vi "Get Alias.vi"(8 "error in (no error)":errorcluster, 11 "Project Action in":refnum<class "Project Action.lvclass">) -> (0 "error out":errorcluster, 2 "Alias":string, 3 "Project Action out":refnum<class "Project Action.lvclass">)   [LabVIEW 2020, in "ProjectBuilder.lvlib" / "Project Action.lvclass"]
uses:
  Project Action.lvclass
  C:/Current projects/WS/LV32.2020..ProjectBuilder/Class/Action/Project Action/Project Action.lvclass
  C:/Current projects/WS/LV32.2020..ProjectBuilder/Interface/Project Action Interface/Project Action Interface.lvclass
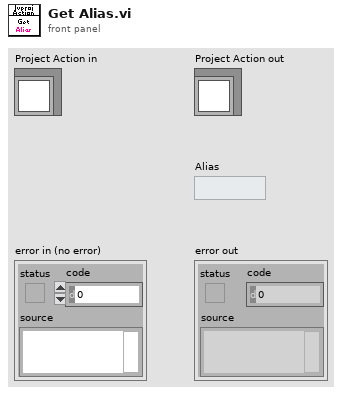
[diagram p1: front panel]
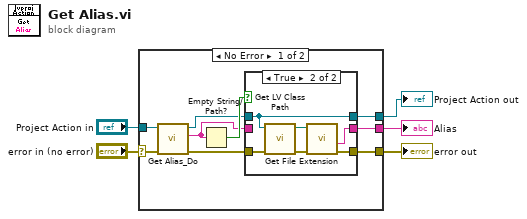
[diagram p0: block diagram]
diagram:
  n1 = case shown="No Error" "error in (no error)" {
    selector: "error in (no error)" -> [w14 w25]
    tunnel: [w7 w25] -> w4
    tunnel: [w9 w24] -> w2
    tunnel: "Project Action in" -> [w13 w24]
    tunnel: [w6 _] -> w1
    frame No Error {
      n2 = call-dynamic "Get Alias_Do.vi"("error in (no error)"=w14, "Project Action in"=w13) -> ("error out"=w8:errorcluster, "Alias"=w11:string, "Project Action out"=w10:refnum<class "Project Action.lvclass">)  [unwired: 7 in]
      n3 = Empty String/Path?(string/path=w11) -> (empty?=w12:bool)
      n4 = case shown="True" w12 {
        tunnel: w11 -> [w15 _]
        tunnel: [w17 w23] -> w9
        tunnel: w10 -> [w17 w23]
        tunnel: [w16 w19] -> w7
        tunnel: w8 -> [w16 w21]
        tunnel: [w15 w18] -> w6
        frame False {
        }
        frame True {
          n5 = call <vilib>:"Get LV Class Path.vi"("error in (no error)"=w21, "object"=w23) -> ("error out"=w20:errorcluster, "class path"=w22:path)  [unwired: 8 in]
          n6 = call <vilib>:"Get File Extension.vi"("error in (no error)"=w20, "file"=w22) -> ("error out"=w19:errorcluster, "filename without extension"=w18:string)  [unwired: 5 in, 3 out]
        }
      }
    }
    frame Error {
    }
  }
  "error out" <- w4
  "Project Action out" <- w2
  "Alias" <- w1
